vi "database1查询.vi"(7 "终止时间":string, 8 "error in (no error)":errorcluster, 9 "table":string, 10 "起始时间":string, 11 "database":string="database1.mdb") -> (0 "error out":errorcluster, 1 "database溢出":bool, 2 "data":string[][](table), 3 "recordset data":variant[][](array[variant]))   [LabVIEW 2016, in "数据传输系统-02.lvlib"]
uses:
  <vilib>/Utility/sysdir.llb/System Directory Type.ctl
  <vilib>/addons/database/Connection.llb/DB Tools Open Connec (String).vi
  <vilib>/addons/database/Connection.llb/Conn Execute.vi
  <vilib>/addons/database/Recordset.llb/Rec Fetch Recordset Data (R).vi
  <vilib>/addons/database/Recordset.llb/Rec Destroy - Connection.vi
  <vilib>/addons/database/_DB Variant To Data/Database Variant To Data.xnode
  <vilib>/addons/database/NI_Database_API.lvlib
panel:
  out "结果字符串":string
  out "仪器代号":string[](array[string])
  out "连接的字符串":string
  out "SQL query":string
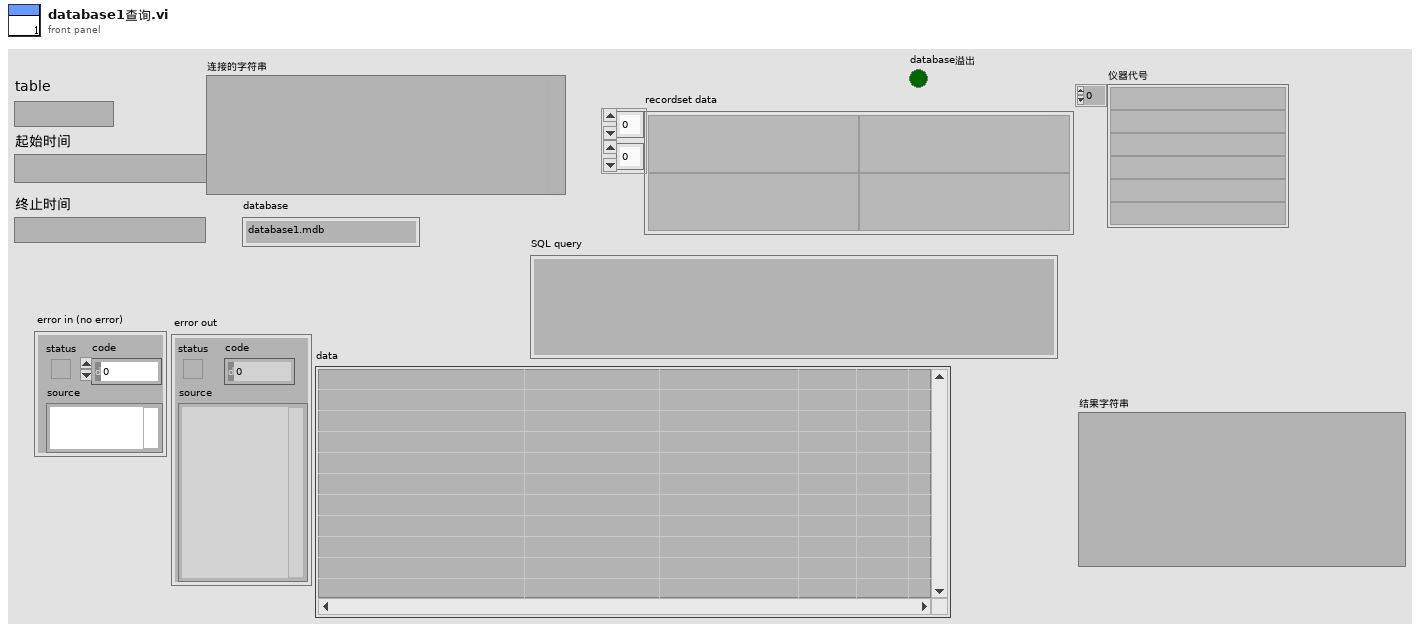
[diagram p1: front panel]
types:
  T1 = typedef "Semaphore RefNum" = refnum<k1>
  T2 = typedef "System Directory Type.ctl" = i32
  T3 = typedef "NI_Database_API.lvlib/Conn ObjectReference.ctl" = refnum<k1>
  T4 = typedef "NI_Database_API.lvlib/Rec ObjectReference.ctl" = refnum<k1>
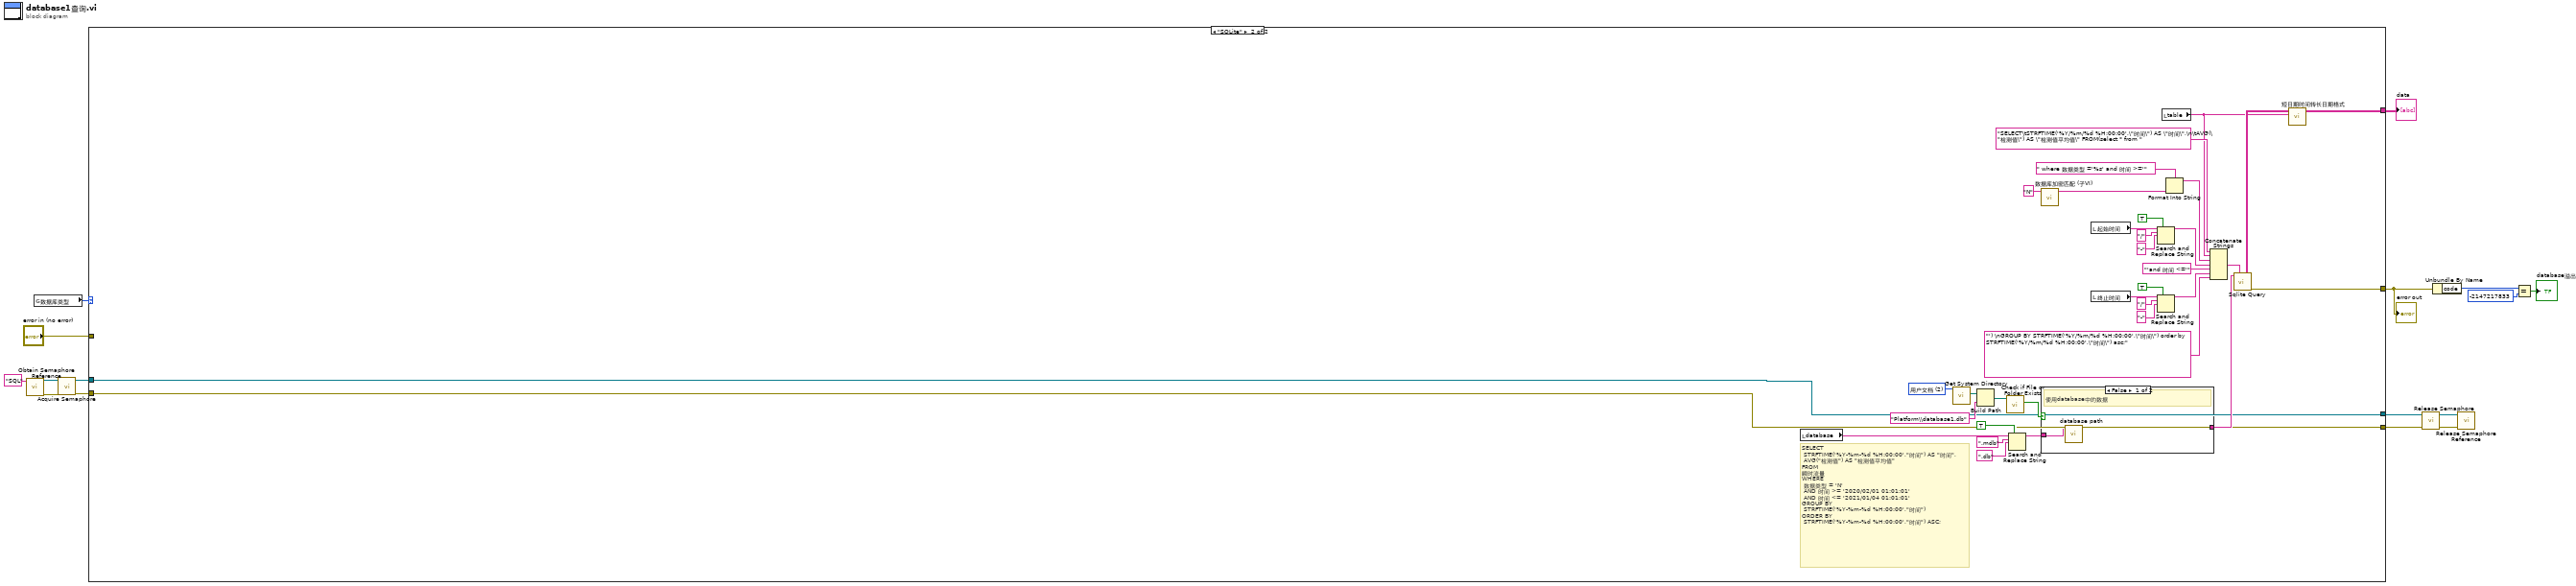
[diagram p0: block diagram]
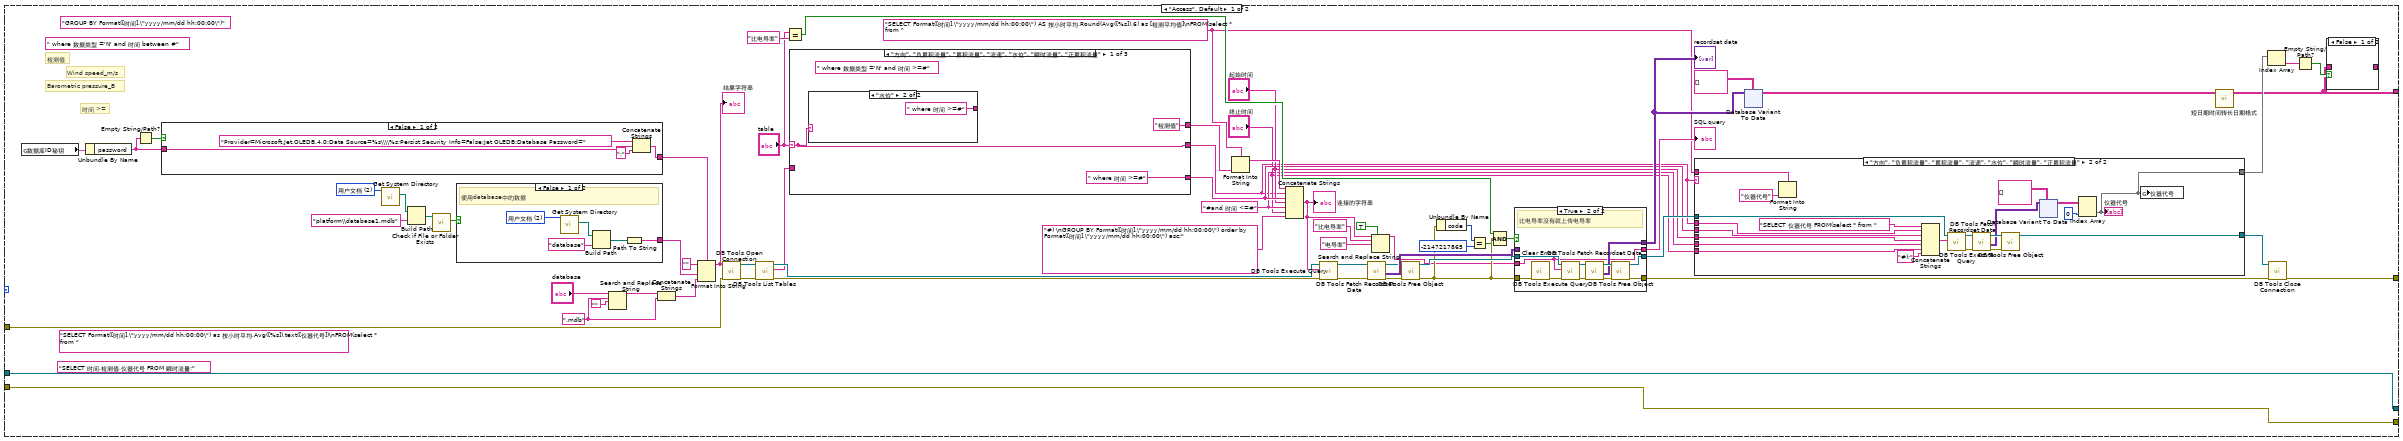
[diagram p2: hidden frame]
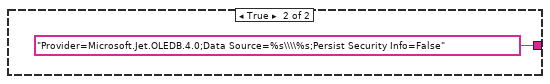
[diagram p5: hidden frame]
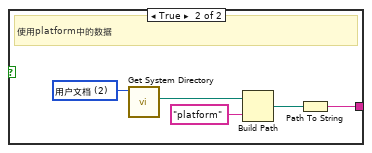
[diagram p7: hidden frame]
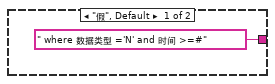
[diagram p8: hidden frame]
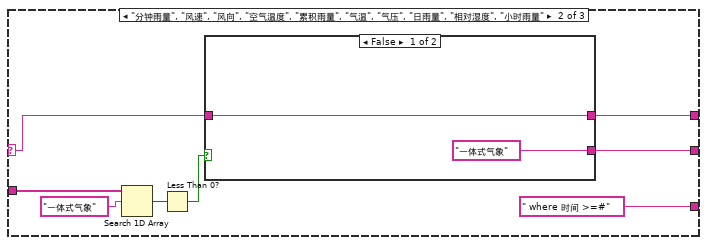
[diagram p9: hidden frame]
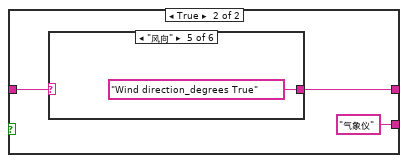
[diagram p10: hidden frame]
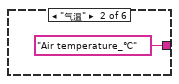
[diagram p12: hidden frame]
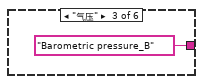
[diagram p13: hidden frame]
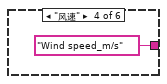
[diagram p14: hidden frame]
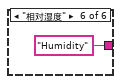
[diagram p15: hidden frame]
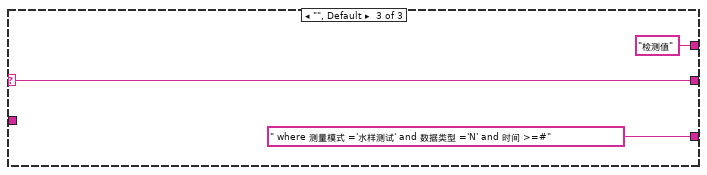
[diagram p16: hidden frame]
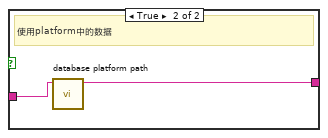
[diagram p17: hidden frame]
diagram:
  n1 = call <vilib>:"Obtain Semaphore Reference.vi"("name (unnamed)"="SQL") -> ("error out"=w7:errorcluster, "semaphore"=w8:T1)  [unwired: 4 in, 1 out]
  n2 = global read "断电保存全局.vi" "数据库类型"() -> (w16:enum16{"Access", "SQLite"})
  n3 = call <vilib>:"Acquire Semaphore.vi"("error in (no error)"=w7, "semaphore"=w8) -> ("error out"=w5:errorcluster, "semaphore out"=w6:T1)  [unwired: 3 in, 1 out]
  n4 = case shown="\"SQLite\"" w16 {
    tunnel: [w49 w261] -> w13
    tunnel: "error in (no error)" -> [w48 _]
    tunnel: [w24 w277] -> w14
    tunnel: w6 -> [w17 w251]
    tunnel: w5 -> [w18 w250]
    tunnel: [w18 w250] -> w2
    tunnel: [w17 w251] -> w1
    frame "Access", Default {
      w29 = "SELECT Format([时间],\"yyyy/mm/dd hh:00:00\") AS 按小时平均,Round(Avg([%s]),6) as [检测平均值]\nFROM(select * from "
      (unwired) "SELECT 时间,检测值,仪器代号 FROM 瞬时流量;" ("连接的字符串")
      w41 = ".mdb" ("搜索字符串")
      (unwired) " where 数据类型 ='N' and 时间 between #"
      w78 = T2 2 items=["用户目录"=0, "用户桌面"=1, "用户文档"=2, "用户应用程序数据"=3, "用户设置"=4, "用户临时目录"=5, "公共文档"=6, "公共应用程序数据"=7, "公共设置"=8, "公共缓存"=13, "系统核心库"=9, "系统安装库"=10, "应用程序文件"=11, "启动盘根目录"=12] ("system directory type")
      (unwired) "GROUP BY Format([时间],\"yyyy/mm/dd hh:00:00\")"
      w34 = "#and 时间 <=#"
      (unwired) "SELECT Format([时间],\"yyyy/mm/dd hh:00:00\") as 按小时平均,Avg([%s]),text([仪器代号])\nFROM(select * from "
      # "时间 >="
      # "Wind speed_m/s"
      # "检测值"
      # "Barometric pressure_B"
      n5 = global read "外部交互全局.vi" "数据库ID秘钥"() -> (w50:cluster{"userID":string, "password":string})
      n6 = Unbundle By Name(w50) -> ("password"=w52:string)
      n7 = Empty String/Path?(string/path=w52) -> (empty?=w25:bool)
      n8 = case shown="False" w25 {
        tunnel: [w194 "Provider=Microsoft.Jet.OLEDB.4.0;Data Source=%s\\\\%s;Persist Security Info=False" ("格式字符串")] -> w51
        tunnel: w52 -> [w193 _]
        frame False {
          n9 = Concatenate Strings("Provider=Microsoft.Jet.OLEDB.4.0;Data Source=%s\\\\%s;Persist Security Info=False;Jet OLEDB:Database Password=" ("格式字符串"), w193, ";" ("字符串")) -> (w194:string)
        }
        frame True {
        }
      }
      n10 = call <vilib>:"Get System Directory.vi"("system directory type"=w78) -> ("system directory"=w79:path)  [unwired: 10 in]
      n11 = Build Path(base path=w79, name or relative path="platform\\database1.mdb" ("condition")) -> (appended path=w77:path)
      n12 = call <vilib>:"Check if File or Folder Exists.vi"("path"=w77) -> ("file or folder exists?"=w75:bool)  [unwired: 8 in, 2 out]
      n13 = case shown="False" w75 {
        tunnel: [w213 w218] -> w74
        frame False {
          w216 = T2 2 items=["用户目录"=0, "用户桌面"=1, "用户文档"=2, "用户应用程序数据"=3, "用户设置"=4, "用户临时目录"=5, "公共文档"=6, "公共应用程序数据"=7, "公共设置"=8, "公共缓存"=13, "系统核心库"=9, "系统安装库"=10, "应用程序文件"=11, "启动盘根目录"=12] ("system directory type")
          # "使用database中的数据"
          n14 = call <vilib>:"Get System Directory.vi"("system directory type"=w216) -> ("system directory"=w215:path)  [unwired: 10 in]
          n15 = Build Path(base path=w215, name or relative path="database" ("condition")) -> (appended path=w217:path)
          n16 = Path To String(path=w217) -> (string=w213:string)
        }
        frame True {
          w222 = T2 2 items=["用户目录"=0, "用户桌面"=1, "用户文档"=2, "用户应用程序数据"=3, "用户设置"=4, "用户临时目录"=5, "公共文档"=6, "公共应用程序数据"=7, "公共设置"=8, "公共缓存"=13, "系统核心库"=9, "系统安装库"=10, "应用程序文件"=11, "启动盘根目录"=12] ("system directory type")
          # "使用platform中的数据"
          n17 = call <vilib>:"Get System Directory.vi"("system directory type"=w222) -> ("system directory"=w221:path)  [unwired: 10 in]
          n18 = Build Path(base path=w221, name or relative path="platform" ("condition")) -> (appended path=w219:path)
          n19 = Path To String(path=w219) -> (string=w218:string)
        }
      }
      n20 = Search and Replace String(input string="database", search string=w41, replace string="") -> (result string=w42:string)  [unwired: 5 in, 3 out]
      n21 = Concatenate Strings(w42, w41) -> (w39:string)
      n22 = Format Into String(format string=w51, initial string="" ("初始字符串"), w74, w39) -> (resulting string=w73:string)  [unwired: 1 in, 1 out]
      "结果字符串" <- w73
      n23 = call-poly <vilib>:"DB Tools Open Connection.vi"("error in (no error)"=w48, "connection information"=w73) -> ("error out"=w23:errorcluster, "connection reference"=w22:T3)  [unwired: 6 in]
      n24 = call <vilib>:"DB Tools List Tables.vi"("error in (no error)"=w23, "connection reference"=w22) -> ("error out"=w20:errorcluster, "tables"=w19:string[], "connection reference out"=w21:T3)  [unwired: 3 in]
      n25 = Equal?(x="table", y="比电导率") -> (x = y?=w68:bool)
      n26 = case shown="\"方向\", \"负累积流量\", \"累积流量\", \"流速\", \"水位\", \"瞬时流量\", \"正累积流量\"" "table" {
        selector: "table" -> [w224 w229 w248]
        tunnel: [" where 时间 >=#" " where 时间 >=#" " where 测量模式 ='水样测试' and 数据类型 ='N' and 时间 >=#"] -> w36
        tunnel: ["检测值" w228 "检测值"] -> w55
        tunnel: [w224 w234 w248] -> w31
        tunnel: w19 -> [_ w233 _]
        frame "方向", "负累积流量", "累积流量", "流速", "水位", "瞬时流量", "正累积流量" {
          (unwired) " where 数据类型 ='N' and 时间 >=#"
          n27 = case shown="\"水位\"" w224 {
            tunnel: [" where 数据类型 ='N' and 时间 >=#" " where 时间 >=#"] -> _
            frame "假", Default {
            }
            frame "水位" {
            }
          }
        }
        frame "分钟雨量", "风速", "风向", "空气温度", "累积雨量", "气温", "气压", "日雨量", "相对湿度", "小时雨量" {
          n28 = Search 1D Array(1D array=w233, element="一体式气象") -> (index of element=w231:i32)  [unwired: 1 in]
          n29 = Less Than 0?(x=w231) -> (x < 0?=w230:bool)
          n30 = case shown="False" w230 {
            tunnel: ["一体式气象" "气象仪"] -> w234
            tunnel: w229 -> [w236 w240]
            tunnel: [w236 w238] -> w228
            frame False {
            }
            frame True {
              n31 = case shown="\"风向\"" w240 {
                selector: w240 -> [w241 _ _ _ _ _]
                tunnel: [w241 "Air temperature_℃" "Barometric pressure_B" "Wind speed_m/s" "Wind direction_degrees True" "Humidity"] -> w238
                frame Default {
                }
                frame "气温" {
                }
                frame "气压" {
                }
                frame "风速" {
                }
                frame "风向" {
                }
                frame "相对湿度" {
                }
              }
            }
          }
        }
        frame "", Default {
        }
      }
      n32 = Format Into String(format string=w29, w55) -> (resulting string=w53:string)  [unwired: 2 in, 1 out]
      n33 = Concatenate Strings(w53, w31, w36, "起始时间", w34, "终止时间", "#) \nGROUP BY Format([时间],\"yyyy/mm/dd hh:00:00\") order by Format([时间],\"yyyy/mm/dd hh:00:00\") asc;" ("字符串")) -> (w38:string)
      "连接的字符串" <- w38
      n34 = call-poly <vilib>:"DB Tools Execute Query.vi"("error in (no error)"=w20, "SQL query"=w38, "connection reference"=w21) -> ("error out"=w66:errorcluster, "recordset reference"=w70:T4)  [unwired: 5 in]
      n35 = call-poly <vilib>:"DB Tools Fetch Recordset Data.vi"("error in (no error)"=w66, "recordset reference"=w70) -> ("error out"=w81:errorcluster, "recordset data"=w71:variant[][], "recordset reference out"=w67:T4)  [unwired: 3 in]
      n36 = Search and Replace String(replace all?=TRUE ("替换全部？(F)"), input string=w38, search string="比电导率" ("搜索字符串"), replace string="电导率" ("替换字符串(\"\")")) -> (result string=w58:string)  [unwired: 4 in, 3 out]
      n37 = call-poly <vilib>:"DB Tools Free Object.vi"("error in (no error)"=w81, "recordset reference"=w67) -> ("error out"=w62:errorcluster, "connection reference"=w65:T3)  [unwired: 8 in]
      n38 = Unbundle By Name(w62) -> ("code"=w64:i32)
      n39 = Equal?(x=w64, y=-2147217865 ("code")) -> (x = y?=w61:bool)
      n40 = Compound Arithmetic op=AND ("复合运算")(w68, w62, w61) -> (w72:bool)
      n41 = case shown="True" w72 {
        tunnel: w58 -> [w198 w202]
        tunnel: w65 -> [w199 w207]
        tunnel: [w199 w203] -> w37
        tunnel: [w201 w205] -> w44
        tunnel: w71 -> [w201 _]
        tunnel: w62 -> [w200 w212]
        tunnel: [w200 w204] -> w45
        tunnel: [w198 w202] -> w56
        frame False {
        }
        frame True {
          # "比电导率没有就上传电导率"
          n42 = call <vilib>:"Clear Errors.vi"("error in (no error)"=w212) -> ("error out"=w206:errorcluster)  [unwired: 5 in, 1 out]
          n43 = call-poly <vilib>:"DB Tools Execute Query.vi"("error in (no error)"=w206, "SQL query"=w202, "connection reference"=w207) -> ("error out"=w208:errorcluster, "recordset reference"=w210:T4)  [unwired: 5 in]
          n44 = call-poly <vilib>:"DB Tools Fetch Recordset Data.vi"("error in (no error)"=w208, "recordset reference"=w210) -> ("error out"=w211:errorcluster, "recordset data"=w205:variant[][], "recordset reference out"=w209:T4)  [unwired: 3 in]
          n45 = call-poly <vilib>:"DB Tools Free Object.vi"("error in (no error)"=w211, "recordset reference"=w209) -> ("error out"=w204:errorcluster, "connection reference"=w203:T3)  [unwired: 8 in]
        }
      }
      "SQL query" <- w56
      "recordset data" <- w44
      n46 = case shown="\"方向\", \"负累积流量\", \"累积流量\", \"流速\", \"水位\", \"瞬时流量\", \"正累积流量\"" w31 {
        tunnel: w37 -> [w83 w100]
        tunnel: w31 -> [_ w99]
        tunnel: w36 -> [_ w98]
        tunnel: "起始时间" -> [_ w97]
        tunnel: w34 -> [_ w96]
        tunnel: "终止时间" -> [_ w95]
        tunnel: [w83 w92] -> w32
        tunnel: w29 -> [_ w87]
        tunnel: [_ w84] -> w28
        frame "假", Default {
        }
        frame "方向", "负累积流量", "累积流量", "流速", "水位", "瞬时流量", "正累积流量" {
          n47 = Format Into String(format string=w87, "仪器代号" ("输入 1")) -> ()  [unwired: 2 in, 2 out]
          n48 = Concatenate Strings("SELECT 仪器代号 FROM(select * from " ("连接的字符串"), w99, w98, w97, w96, w95, "#);" ("连接的字符串")) -> (w93:string)
          n49 = call-poly <vilib>:"DB Tools Execute Query.vi"("SQL query"=w93, "connection reference"=w100) -> ("error out"=w104:errorcluster, "recordset reference"=w102:T4)  [unwired: 6 in]
          n50 = call-poly <vilib>:"DB Tools Fetch Recordset Data.vi"("error in (no error)"=w104, "recordset reference"=w102) -> ("error out"=w101:errorcluster, "recordset data"=w91:variant[][], "recordset reference out"=w103:T4)  [unwired: 3 in]
          n51 = call-poly <vilib>:"DB Tools Free Object.vi"("error in (no error)"=w101, "recordset reference"=w103) -> ("connection reference"=w92:T3)  [unwired: 8 in, 1 out]
          n52 = xnode "Database Variant To Data"("database variant"=w91, "type"=string[][] []) -> ("data"=w89:string[][])  [unwired: 1 in, 1 out]
          n53 = Index Array(array=w89, index (col)=0 ("禁用的索引 (列)")) -> (element=w84:string[])  [unwired: 1 in]
          "仪器代号" <- w84
          n54 = global write "全局 所有参数.vi" "仪器代号"(w84) -> ()
        }
      }
      n55 = xnode "Database Variant To Data"("database variant"=w44, "type"=string[][] []) -> ("data"=w46:string[][])  [unwired: 1 in, 1 out]
      n56 = call "短日期时间转长日期格式.vi"("data"=w46) -> ("输出数组"=w24:string[][])  [unwired: 10 in]
      n57 = Index Array(array=w28) -> (element=w27:string)  [unwired: 1 in]
      n58 = call <vilib>:"DB Tools Close Connection.vi"("error in (no error)"=w45, "connection reference"=w32) -> ("error out"=w49:errorcluster)  [unwired: 5 in]
      n59 = Empty String/Path?(string/path=w27) -> (empty?=w26:bool)
      n60 = case shown="False" w26 {
        tunnel: w24 -> [_ w82]
        tunnel: [_ w82] -> _
        frame False {
        }
        frame True {
        }
      }
    }
    frame "SQLite" {
      w281 = T2 2 items=["用户目录"=0, "用户桌面"=1, "用户文档"=2, "用户应用程序数据"=3, "用户设置"=4, "用户临时目录"=5, "公共文档"=6, "公共应用程序数据"=7, "公共设置"=8, "公共缓存"=13, "系统核心库"=9, "系统安装库"=10, "应用程序文件"=11, "启动盘根目录"=12] ("system directory type")
      # "SELECT\n\tSTRFTIME('%Y-%m-%d %H:00:00',\"时间\") AS \"时间\",\n\tAVG(\"检测值\") AS \"检测值平均值\"\nFROM\n瞬时流量 \nWHERE\n\t数据类型 = 'N' \n\tAND 时间 >= '2020/02/01 01:01:01' \n\tAND 时间 <= '2021/01/04 01:01:01' \nGROUP BY\n\tSTRFTIME('%Y-%m-%d %H:00:00',\"时间\")\nORDER BY\n\tSTRFTIME('%Y-%m-%d %H:00:00',\"时间\") ASC;"
      n61 = local read "database"() -> (w262:string)
      n62 = call <vilib>:"Get System Directory.vi"("system directory type"=w281) -> ("system directory"=w280:path)  [unwired: 10 in]
      n63 = Build Path(base path=w280, name or relative path="Platform\\database1.db" ("condition")) -> (appended path=w282:path)
      n64 = call <vilib>:"Check if File or Folder Exists.vi"("path"=w282) -> ("file or folder exists?"=w284:bool)  [unwired: 8 in, 2 out]
      n65 = Search and Replace String(replace all?=TRUE ("替换全部？(F)"), input string=w262, search string=".mdb" ("搜索字符串"), replace string=".db" ("替换字符串(\"\")")) -> (result string=w253:string)  [unwired: 4 in, 3 out]
      n66 = call "数据库加密匹配 (子VI).vi"("输入参数"="N") -> ("Encoded String"=w255:string)  [unwired: 10 in]
      n67 = case shown="False" w284 {
        tunnel: [w285 w287] -> w252
        tunnel: w253 -> [w286 w288]
        frame False {
          # "使用database中的数据"
          n68 = call "database path.vi"("database"=w286) -> ("Path out"=w285:string)  [unwired: 9 in, 1 out]
        }
        frame True {
          # "使用platform中的数据"
          n69 = call "database platform path.vi"("database"=w288) -> ("Path out"=w287:string)  [unwired: 10 in]
        }
      }
      n70 = local read "起始时间"() -> (w269:string)
      n71 = local read "终止时间"() -> (w267:string)
      n72 = Search and Replace String(replace all?=TRUE ("替换全部？(F)"), input string=w269, search string="/" ("搜索字符串"), replace string="-" ("替换字符串(\"\")")) -> (result string=w268:string)  [unwired: 4 in, 3 out]
      n73 = Search and Replace String(replace all?=TRUE ("替换全部？(F)"), input string=w267, search string="/" ("搜索字符串"), replace string="-" ("替换字符串(\"\")")) -> (result string=w266:string)  [unwired: 4 in, 3 out]
      n74 = local read "table"() -> (w259:string)
      n75 = Format Into String(format string=" where 数据类型 ='%s' and 时间 >='", w255) -> (resulting string=w257:string)  [unwired: 2 in, 1 out]
      n76 = Concatenate Strings("SELECT\tSTRFTIME('%Y/%m/%d %H:00:00',\"时间\") AS \"时间\",\n\tAVG(\"检测值\") AS \"检测值平均值\" FROM(select * from ", w259, w257, w268, "'and 时间 <='", w266, "') \nGROUP BY STRFTIME('%Y/%m/%d %H:00:00',\"时间\") order by STRFTIME('%Y/%m/%d %H:00:00',\"时间\") asc;" ("字符串")) -> (w254:string)
      n77 = call "Sqlite Query.vi"("DB Path"=w252, "SQL Query"=w254) -> ("Results"=w260:string[][], "error out"=w261:errorcluster)  [unwired: 11 in, 1 out]
      n78 = call "短日期时间转长日期格式.vi"("table输入"=w259, "data"=w260) -> ("输出数组"=w277:string[][])  [unwired: 9 in]
    }
  }
  "error out" <- w13
  "data" <- w14
  n79 = call <vilib>:"Release Semaphore.vi"("error in (no error)"=w2, "semaphore"=w1) -> ("error out"=w3:errorcluster, "semaphore out"=w4:T1)  [unwired: 4 in]
  n80 = Unbundle By Name(w13) -> ("code"=w12:i32)
  n81 = call <vilib>:"Release Semaphore Reference.vi"("error in (no error)"=w3, "semaphore"=w4) -> ()  [unwired: 8 in, 2 out]
  n82 = Equal?(x=w12, y=-2147217833 ("code")) -> (x = y?=→"database溢出":bool)
